vi "SAVE_Punching_Bag.vi"() -> ()   [LabVIEW 2017]
panel:
  in  "name or relative path":string
  out "Sine":dynamicdata(graph)
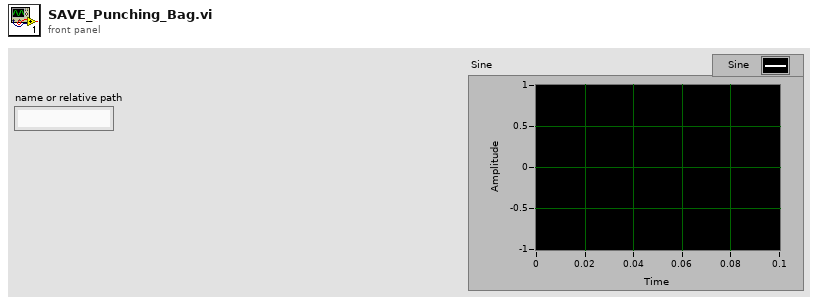
[diagram p1: front panel]
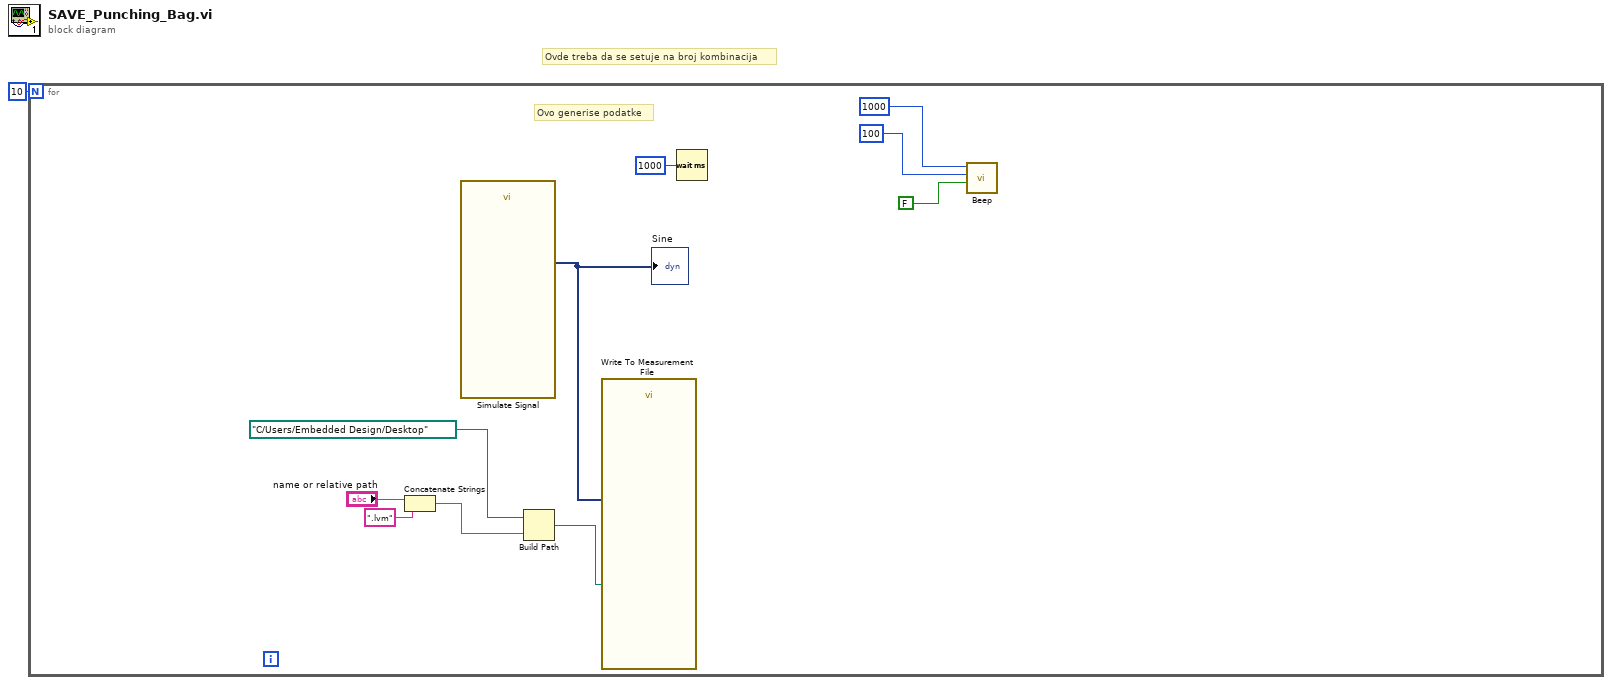
[diagram p0: block diagram]
diagram:
  # "Ovde treba da se setuje na broj kombinacija"
  n1 = for {
    N: 10 -> [_]
    # "Ovo generise podatke"
    n2 = Concatenate Strings("name or relative path", ".lvm" ("string")) -> (w5:string)
    n3 = call "Simulate Signal"() -> ("Sine"=w10:dynamicdata)  [unwired: 14 in, 1 out]
    "Sine" <- w10
    n4 = Build Path(base path=path "C:/Users/Embedded Design/Desktop", name or relative path=w5) -> (appended path=w3:path)
    n5 = call "Write To Measurement File"("Signals"=w10, "Filename"=w3) -> ()  [unwired: 15 in, 3 out]
    n6 = Wait (ms)(milliseconds to wait=u32 1000) -> ()  [unwired: 1 out]
    n7 = call <vilib>:"Beep.vi"("use system alert? (T)"=FALSE, "duration (msec)"=u32 100, "frequency (Hz)"=u32 1000) -> ()  [unwired: 9 in]
  }
